vi "A.vi"() -> ()   [LabVIEW 2010]
panel:
  out "loop counter":i32
  in  "stop":bool
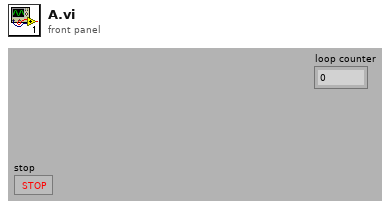
[diagram p1: front panel]
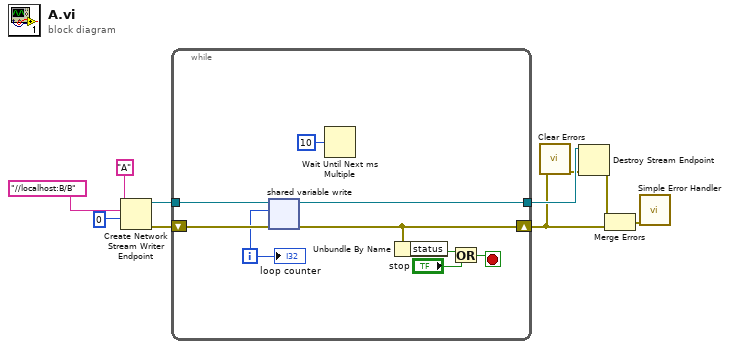
[diagram p0: block diagram]
diagram:
  n1 = Create Network Stream Writer Endpoint(9:0, 10:"//localhost:B/B" ("reader url"), 11:"A" ("writer name")) -> (0:w10:errorcluster, 3:w9:refnum<k21>)  [unwired: 3 in]
  n2 = while {
    shift-right: [w15] -> w2
    shift-left: w10 -> [w18]
    tunnel: w9 -> [w17]
    tunnel: [w11] -> w5
    i -> [w16]
    stop <- w12 stop-if-true
    n3 = shared-variable-write(w17, w18, w16) -> (w11:refnum<k21>, w15:errorcluster)  [unwired: 1 in, 1 out]
    n4 = Wait Until Next ms Multiple(millisecond multiple=u32 10) -> ()  [unwired: 1 out]
    n5 = Unbundle By Name(w15) -> ("status"=w14:bool)
    n6 = Or(x=w14, y="stop") -> (x .or. y?=w12:bool)
    "loop counter" <- w16
  }
  n7 = call <vilib>:"Clear Errors.vi"("error in (no error)"=w2) -> ("error out"=w4:errorcluster)  [unwired: 6 in]
  n8 = Destroy Stream Endpoint(8:w4, 11:w5) -> (0:w3:errorcluster)
  n9 = Merge Errors(w3, w2) -> (w1:errorcluster)
  n10 = call <vilib>:"Simple Error Handler.vi"("error in (no error)"=w1) -> ()  [unwired: 4 in, 5 out]
